vi "Force Table Number 2 Dataset Id.vi"(4 "Table Number":i32) -> (0 "Dataset Source":T1, 1 "Dataset Type":T2)   [LabVIEW 2009]
uses:
  Global Data/Transactions/Dataset Type.ctl
  Global Data/Transactions/Dataset Source.ctl
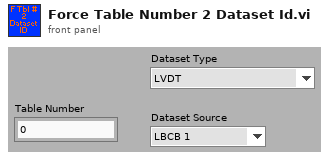
[diagram p1: front panel]
types:
  T1 = typedef "Dataset Source.ctl" = enum16{"LBCB 1", "LBCB 2", "Combined", "External Sensors"}
  T2 = typedef "Dataset Type.ctl" = enum16{"LVDT", "Load Cell", "Actuator Command", "Servo Error", "Displacement Command", "Displacement", "Force"}
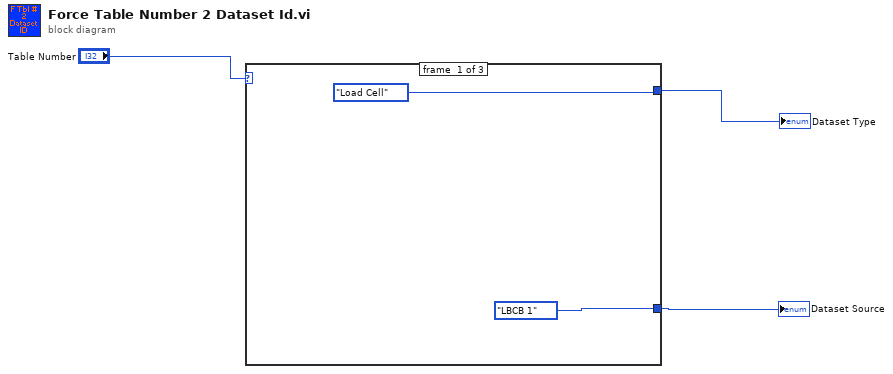
[diagram p0: block diagram]
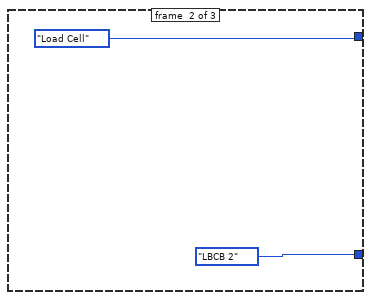
[diagram p2: hidden frame]
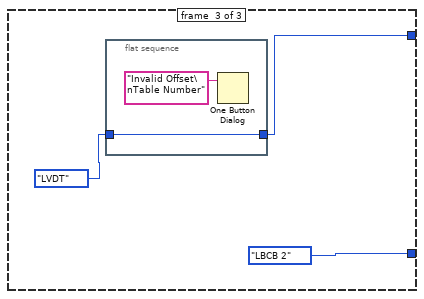
[diagram p3: hidden frame]
diagram:
  n1 = case shown="1" "Table Number" {
    tunnel: [Dataset_Source."LBCB 1" ("Dataset Source") Dataset_Source."LBCB 2" ("Dataset Source") Dataset_Source."LBCB 2" ("Dataset Source")] -> w2
    tunnel: [Dataset_Type."Load Cell" ("Dataset Type") Dataset_Type."Load Cell" ("Dataset Type") w8] -> w3
    frame #0 {
    }
    frame #1 {
    }
    frame #2 {
      n2 = flat-sequence {
        tunnel: Dataset_Type."LVDT" ("Dataset Type") -> [w12]
        tunnel: [w12] -> w8
        frame #0 {
          n3 = One Button Dialog(message="Invalid Offset\nTable Number") -> ()  [unwired: 1 in, 1 out]
        }
      }
    }
  }
  "Dataset Type" <- w3
  "Dataset Source" <- w2
